vi "delete.vi"(2 "future event?":bool=TRUE, 3 "Value":i32[](array[numeric]), 4 "ItemNames in":string[][](array[string])) -> (0 "val(sgnl)":i32[](array[numeric]), 1 "ItemNames out":string[][](array[string]))   [LabVIEW 2020]
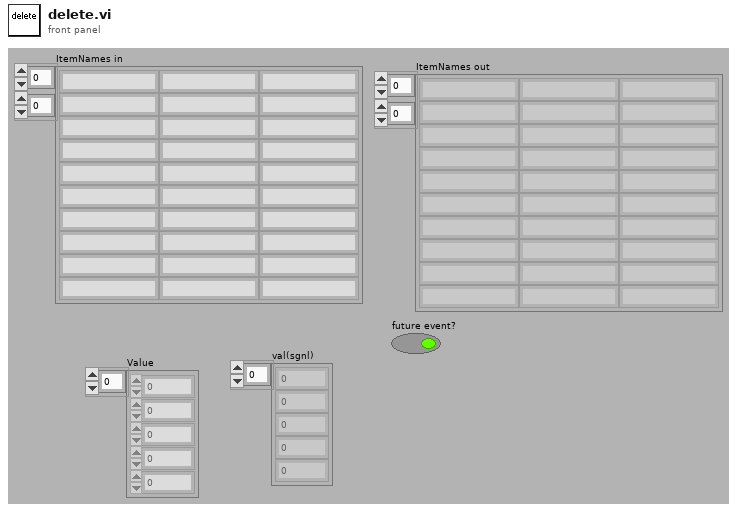
[diagram p1: front panel]
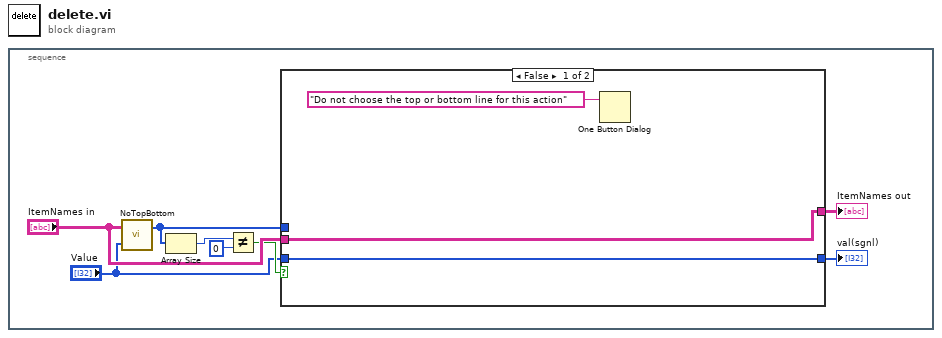
[diagram p0: block diagram]
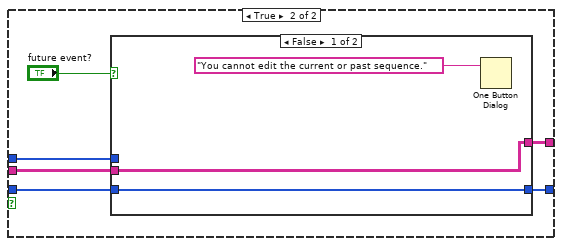
[diagram p2: hidden frame]
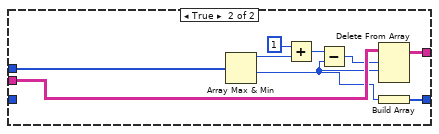
[diagram p3: hidden frame]
diagram:
  n1 = stacked-sequence {
    frame #0 {
      n2 = call "NoTopBottom.vi"("Value in"="Value", "ItemNames in"="ItemNames in") -> ("Value out"=w2:i32[])  [unwired: 1 out]
      n3 = Array Size(array=w2) -> (size(s)=w3:i32)
      n4 = Not Equal?(x=w3, y=0) -> (x != y?=w4:bool)
      n5 = case shown="False" w4 {
        tunnel: [w11 w16] -> w8
        tunnel: [w9 w15] -> w7
        tunnel: "ItemNames in" -> [w11 w14]
        tunnel: w2 -> [_ w13]
        tunnel: "Value" -> [w9 w12]
        frame False {
          n6 = One Button Dialog(message="Do not choose the top or bottom line for this action") -> ()  [unwired: 1 in, 1 out]
        }
        frame True {
          n7 = case shown="False" "future event?" {
            tunnel: w14 -> [w20 w26]
            tunnel: [w20 w25] -> w16
            tunnel: w13 -> [_ w24]
            tunnel: [w18 w23] -> w15
            tunnel: w12 -> [w18 _]
            frame False {
              n8 = One Button Dialog(message="You cannot edit the current or past sequence.") -> ()  [unwired: 1 in, 1 out]
            }
            frame True {
              n9 = Array Max & Min(array=w24) -> (max value=w28:i32, min value=w21:i32)  [unwired: 2 out]
              n10 = Add(x=1, y=w28) -> (x+y=w29:i32)
              n11 = Subtract(x=w29, y=w21) -> (x-y=w22:i32)
              n12 = Delete From Array(array=w26, length=w22, index (row)=w21) -> (array with subset deleted=w25:string[][])  [unwired: 1 in, 1 out]
              n13 = Build Array(w21) -> (w23:i32[])
            }
          }
        }
      }
      "ItemNames out" <- w8
      "val(sgnl)" <- w7
    }
  }
